vi "ValidateOwner.vi"(8 "error in (no error)":errorcluster, 10 "Shared Key":string, 11 "SMO in":refnum<class "SMO.lvclass">) -> (0 "error out":errorcluster, 1 "not set":bool, 2 "key matched":bool, 3 "SMO out":refnum<class "SMO.lvclass">)   [LabVIEW 2013, in "SMO.lvclass"]
uses:
  SMO.lvclass
  SMO.lvclass/SMO.ctl
  Support/Attribute.Owner/Attribute.Owner.lvclass
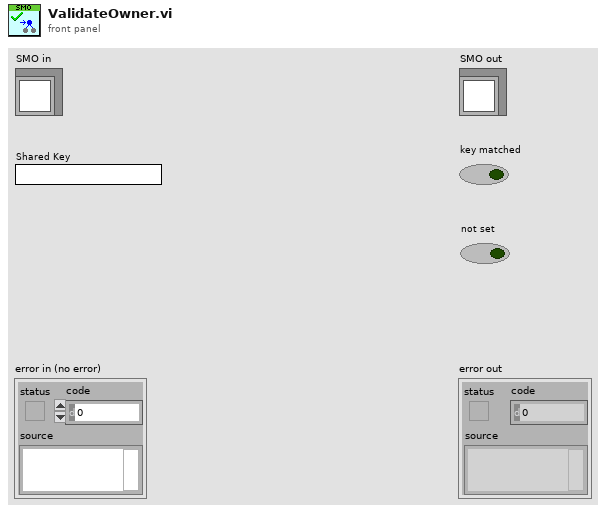
[diagram p1: front panel]
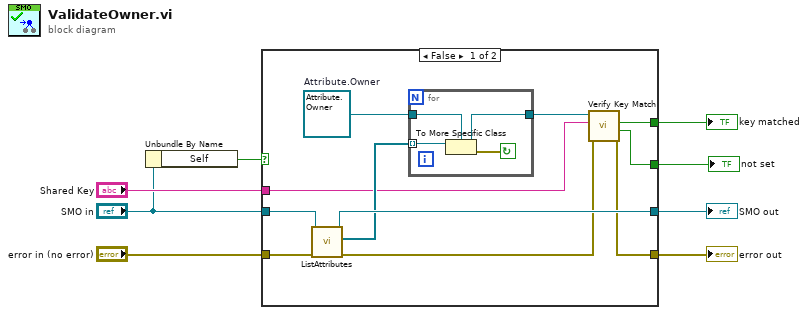
[diagram p0: block diagram]
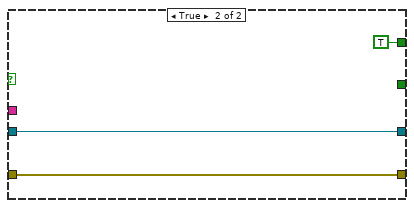
[diagram p2: hidden frame]
diagram:
  n1 = Unbundle By Name("SMO in") -> ("Self"=w2:bool)
  n2 = case shown="False" w2 {
    tunnel: "error in (no error)" -> [w19 w24]
    tunnel: [w18 w25] -> w7
    tunnel: "Shared Key" -> [w14 _]
    tunnel: [w12 w24] -> w5
    tunnel: [w11 TRUE ("key matched")] -> w4
    tunnel: "SMO in" -> [w10 w25]
    tunnel: [w9 _] -> w1
    frame False {
      w16 = refnum<class "Attribute.Owner.lvclass"> refnum  # Attribute.Owner
      n3 = call "ListAttributes.vi"("error in (no error)"=w19, "SMO in"=w10) -> ("error out"=w13:errorcluster, "[Attributes]"=w17:refnum<class "Attribute.lvclass">[], "SMO out"=w18:refnum<class "SMO.lvclass">)  [unwired: 7 in]
      n4 = for {
        tunnel: w17 -> [w23] mode=indexing
        tunnel: w16 -> [w22]
        tunnel: [w20] -> w15
        stop <- w21 continue-if-true
        n5 = To More Specific Class(target class=w22, reference=w23) -> (specific class reference=w20:refnum<class "Attribute.Owner.lvclass">, error out=w21:errorcluster)  [unwired: 1 in]
      }
      n6 = call "Verify Key Match.vi"("error in (no error)"=w13, "Shared Key"=w14, "Attribute.Owner in"=w15) -> ("error out"=w12:errorcluster, "not set"=w9:bool, "key matched"=w11:bool)  [unwired: 5 in, 1 out]
    }
    frame True {
    }
  }
  "error out" <- w5
  "SMO out" <- w7
  "key matched" <- w4
  "not set" <- w1
